vi "Intake Rollers.vi"   [LabVIEW 2014]
uses:
  Begin/Global RefNums.vi
  Begin/Global Variables.vi
  <vilib>/Rock Robotics/WPI/Solenoid/Deprecated/WPI_SolenoidSetBool.vi
types:
  T1 = typedef "WPI_MotorControlDeviceRef.ctl" = cluster{"DeviceStatus":errorcluster, "Type":T2, "PWM":cluster{"Controller":T3, "PWM Channel":T4, "DeadBand":T5}, "CAN":cluster{"Device Number":u8, "Control Mode":T6, "Semaphore":T7, "Max Vout":dbl, "TalonSRX Control Mode":T8}, "Invert":bool, "TransformRef":T9, "InvTransformRef":T9}
  T2 = typedef "WPI_MotorControlType.ctl" = enum16{"PWM", "CAN", "CANTalonSRX"}
  T3 = typedef "FPGA_TypedefDigitalModule.ctl" = enum16{"Controller 1"}
  T4 = typedef "FPGA_DIOPWMChannel.ctl" = enum8{"PWM 0", "PWM 1", "PWM 2", "PWM 3", "PWM 4", "PWM 5", "PWM 6", "PWM 7", "PWM 8", "PWM 9", "PWM MXP 0", "PWM MXP 1", "PWM MXP 2", "PWM MXP 3", "PWM MXP 4", "PWM MXP 5", "PWM MXP 6", "PWM MXP 7", "PWM MXP 8", "PWM MXP 9", "Invalid"}
  T5 = typedef "WPI_PWMDeadband.ctl" = cluster{"Name":string, "maxPositivePwm":i32, "minPositivePwm":i32, "centerPwm":i32, "maxNegativePwm":i32, "minNegativePwm":i32, "angularRange":u16}
  T6 = typedef "WPI_CANJaguar_ControlMode.ctl" = enum8{"Percent VBus", "Current", "Speed", "Position", "Voltage"}
  T7 = typedef "Semaphore RefNum" = refnum<k1>
  T8 = typedef "WPI_CANTalonSRX_APIControlMode.ctl" = enum8{"Percent VBus", "Speed", "Position", "Slave", "Unchanged / Invalid"}
  T9 = typedef "WPI_PWMTransform_ConPane.ctl" = refnum<vi>
  T10 = typedef "WPI_SolenoidDevRef.ctl" = cluster{"DevStatus":errorcluster, "Pneumatics Control Module":u8, "Forward Solenoid Channel":T11, "Reverse Solenoid Channel":T11}
  T11 = typedef "WPI_SolenoidChannel.ctl" = enum8{"Solenoid 0", "Solenoid 1", "Solenoid 2", "Solenoid 3", "Solenoid 4", "Solenoid 5", "Solenoid 6", "Solenoid 7", "Invalid"}
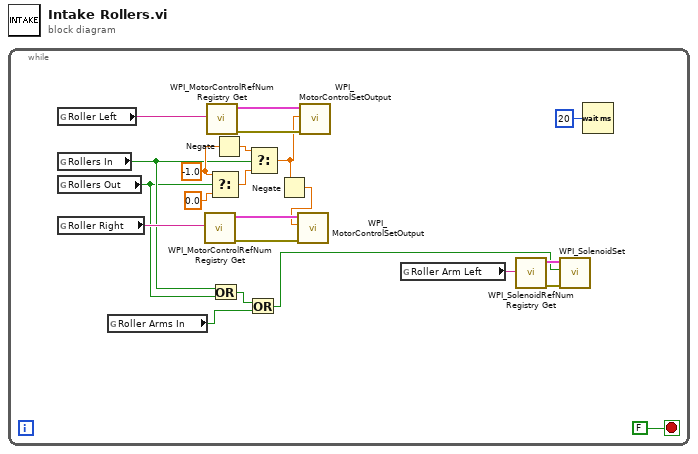
[diagram p0: block diagram]
diagram:
  n1 = while {
    stop <- FALSE stop-if-true
    w13 = -1.0 ("t")
    n2 = global read "Global RefNums.vi" "Roller Left"() -> (w20:string)
    n3 = global read "Global Variables.vi" "Rollers In"() -> (w10:bool)
    n4 = global read "Global Variables.vi" "Rollers Out"() -> (w9:bool)
    n5 = global read "Global RefNums.vi" "Roller Right"() -> (w19:string)
    n6 = global read "Global Variables.vi" "Roller Arms In"() -> (w7:bool)
    n7 = call <vilib>:"WPI_MotorControlRefNum Registry Get.vi"("refnum name"=w19) -> ("error out"=w17:errorcluster, "MotorControlDevRef"=w18:T1)  [unwired: 9 in]
    n8 = call <vilib>:"WPI_MotorControlRefNum Registry Get.vi"("refnum name"=w20) -> ("error out"=w22:errorcluster, "MotorControlDevRef"=w21:T1)  [unwired: 9 in]
    n9 = Select(t=w13, s=w9, f=0.0) -> (s? t:f=w16:dbl)
    n10 = Or(x=w10, y=w9) -> (x .or. y?=w8:bool)
    n11 = Negate(x=w13) -> (-x=w14:dbl)
    n12 = Or(x=w8, y=w7) -> (x .or. y?=w3:bool)
    n13 = Select(t=w14, s=w10, f=w16) -> (s? t:f=w12:dbl)
    n14 = Negate(x=w12) -> (-x=w11:dbl)
    n15 = call <vilib>:"WPI_MotorControlSetOutput.vi"("error in (no error)"=w17, "Output"=w11, "MotorControlDevRef"=w18) -> ()  [unwired: 6 in, 3 out]
    n16 = call <vilib>:"WPI_MotorControlSetOutput.vi"("error in (no error)"=w22, "Output"=w12, "MotorControlDevRef"=w21) -> ()  [unwired: 6 in, 3 out]
    n17 = global read "Global RefNums.vi" "Roller Arm Left"() -> (w4:string)
    n18 = call <vilib>:"WPI_SolenoidRefNum Registry Get.vi"("refnum name"=w4) -> ("error out"=w6:errorcluster, "SolenoidDevRef"=w5:T10)  [unwired: 9 in]
    n19 = call-poly <vilib>:"WPI_SolenoidSet.vi"("error in (no error)"=w6, "Value"=w3, "SolenoidDevRef"=w5) -> ()  [unwired: 7 in, 2 out]
    n20 = Wait (ms)(milliseconds to wait=u32 20) -> ()  [unwired: 1 out]
  }
